vi "Read Encoder Value.vi"(0 "class data in":refnum<class "MB_ENGINE.lvclass">, 1 "init":bool, 11 "error in (no error)":errorcluster) -> (4 "class data out":refnum<class "MB_ENGINE.lvclass">, 6 "type":u16, 8 "Encoder":i32, 10 "Angel (rad)":dbl, 15 "error out":errorcluster)   [LabVIEW 2019, in "MB_ENGINE.lvclass"]
uses:
  MB_ENGINE.lvclass
  MB_ENGINE.lvclass/MB_ENGINE.ctl
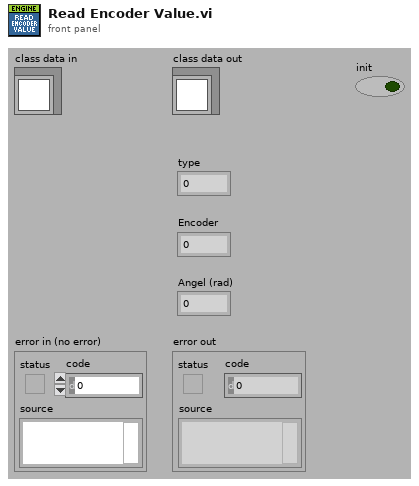
[diagram p1: front panel]
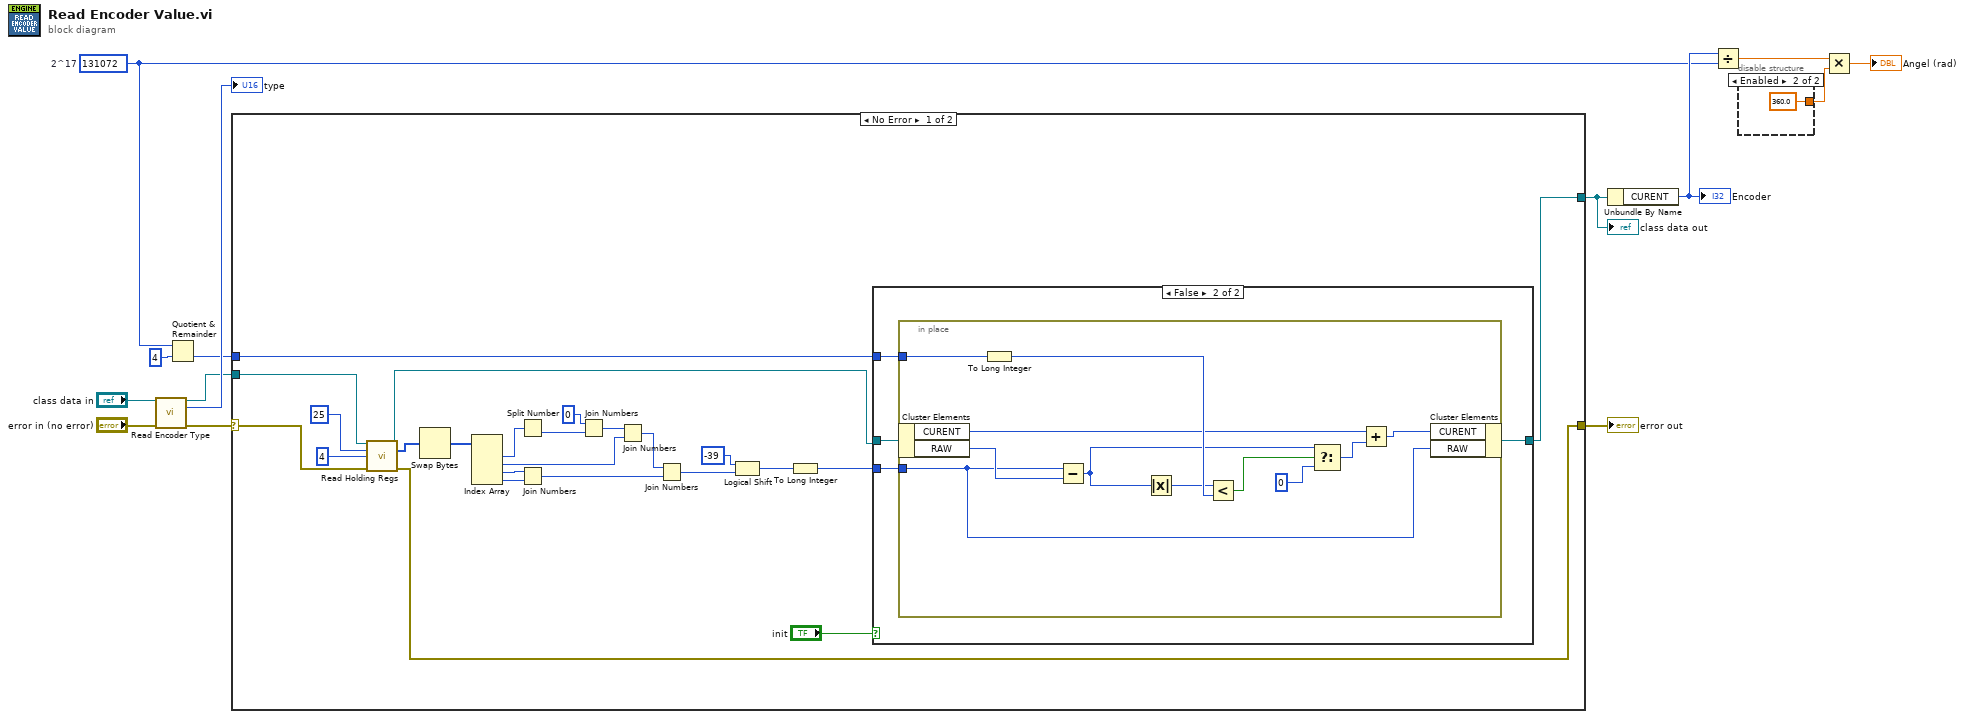
[diagram p0: block diagram]
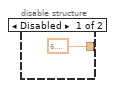
[diagram p2: hidden frame]
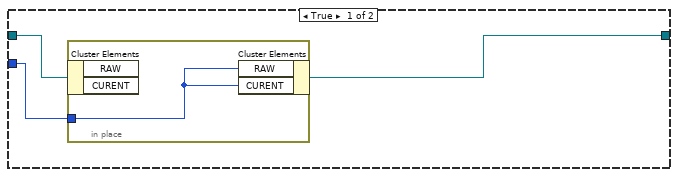
[diagram p3: hidden frame]
diagram:
  w4 = u32 131072  # 2^17
  n1 = call-dynamic "Read Encoder Type.vi"("class data in"="class data in", "error in (no error)"="error in (no error)") -> ("class data out"=w2:refnum<class "MB_ENGINE.lvclass">, "type"=→"type":u16, "error out"=w9:errorcluster)  [unwired: 11 in]
  n2 = Quotient & Remainder(x=w4, y=u32 4) -> (floor(x/y)=w1:u32)  [unwired: 1 out]
  n3 = case shown="No Error" w9 {
    selector: w9 -> [w22 w59]
    tunnel: [w38 w59] -> w14
    tunnel: w2 -> [w18 w58]
    tunnel: [w15 w58] -> w12
    tunnel: w1 -> [w20 _]
    frame No Error {
      n4 = call-dynamic "Read Holding Regs.vi"("reference in"=w18, "starting address"=u16 25, "number of inputs"=u16 4, "error in (no error)"=w22) -> ("reference out"=w16:refnum<class "MB_ENGINE.lvclass">, "register values"=w17:u16[], "error out"=w38:errorcluster)  [unwired: 9 in]
      n5 = Swap Bytes(anything=w17) -> (byte swapped=w34:u16[])
      n6 = Index Array(array=w34) -> (element #1=w26:u16, element #2=w35:u16, element #3=w33:u16, element #4=w32:u16)  [unwired: 4 in]
      n7 = Split Number(x=w26) -> (lo(x)=w25:u8)  [unwired: 1 out]
      n8 = Join Numbers(hi=w33, lo=w32) -> ((hi.lo)=w31:u32)
      n9 = Join Numbers(hi=u8 0, lo=w25) -> ((hi.lo)=w23:u16)
      n10 = Join Numbers(hi=w23, lo=w35) -> ((hi.lo)=w30:u32)
      n11 = Join Numbers(hi=w30, lo=w31) -> ((hi.lo)=w28:u64)
      n12 = Logical Shift(y=i16 -39, x=w28) -> (x << y=w27:u64)
      n13 = To Long Integer(number=w27) -> (32bit integer=w19:i32)
      n14 = case shown="False" "init" {
        tunnel: w16 -> [w41 w46]
        tunnel: w19 -> [w40 w45]
        tunnel: [w39 w44] -> w15
        tunnel: w20 -> [_ w43]
        frame True {
          n15 = in-place {
            in-place-border: w40 -> [w42]
            n16 = in-place-cluster #1(w41) -> ()  [unwired: 2 out]
            n17 = in-place-cluster #1("RAW"=w42, "CURENT"=w42) -> (w39:refnum<class "MB_ENGINE.lvclass">)
          }
        }
        frame False {
          n18 = in-place {
            in-place-border: w45 -> [w52]
            in-place-border: w43 -> [w57]
            n19 = in-place-cluster #2(w46) -> ("CURENT"=w51:i32, "RAW"=w55:i32)
            n20 = To Long Integer(number=w57) -> (32bit integer=w56:i32)
            n21 = Subtract(x=w52, y=w55) -> (x-y=w50:i32)
            n22 = Absolute Value(x=w50) -> (abs(x)=w54:i32)
            n23 = Less?(x=w54, y=w56) -> (x < y?=w53:bool)
            n24 = Select(t=w50, s=w53, f=0) -> (s? t:f=w48:i32)
            n25 = Add(x=w51, y=w48) -> (x+y=w47:i32)
            n26 = in-place-cluster #2("CURENT"=w47, "RAW"=w52) -> (w44:refnum<class "MB_ENGINE.lvclass">)
          }
        }
      }
    }
    frame Error {
    }
  }
  "error out" <- w14
  "class data out" <- w12
  n27 = Unbundle By Name(w12) -> ("CURENT"=w6:i32)
  "Encoder" <- w6
  n28 = Divide(x=w6, y=w4) -> (x/y=w5:dbl)
  n29 = disable-structure shown="Enabled" {
    disable-tunnel: [6.283185307179586 360.0] -> w8
    frame Disabled {
    }
    frame Enabled {
    }
  }
  n30 = Multiply(x=w5, y=w8) -> (x*y=→"Angel (rad)":dbl)
